vi "LoggingSpecificationDocument SetTestProperty.vi"(6 "contextId":T1, 8 "error in":errorcluster, 9 "timeout (ms)":i32=-1, 10 "Request Data":T3, 11 "gRPC ID":T1) -> (0 "error out":errorcluster, 2 "Response Data":T2, 3 "gRPC ID out":T1)   [LabVIEW 2020, in "FlexLogger_client.lvlib"]
uses:
  FlexLogger_client.lvlib
  <vilib>/gRPC/LabVIEW gRPC Library/Shared/grpcId.ctl
  RPC Messages/flexlogger_SetTestPropertyRequest.ctl
  RPC Messages/flexlogger_ElementIdentifier.ctl
  RPC Messages/flexlogger_TestProperty.ctl
  RPC Messages/flexlogger_SetTestPropertyResponse.ctl
  14035477-4c25-4107-8ed5-d0c4ef420ce5.vi
  <vilib>/gRPC/LabVIEW gRPC Library/Shared/TranslateGrpcError.vi
  <vilib>/gRPC/LabVIEW gRPC Library/Shared/Wait On Occurence.vi
  <vilib>/gRPC/LabVIEW gRPC Library/Server API/Server/Get Server DLL Path.vi
  <vilib>/Utility/error.llb/Error Cluster From Error Code.vi
  <vilib>/gRPC/LabVIEW gRPC Library/grpc-lvsupport-release.lvlib
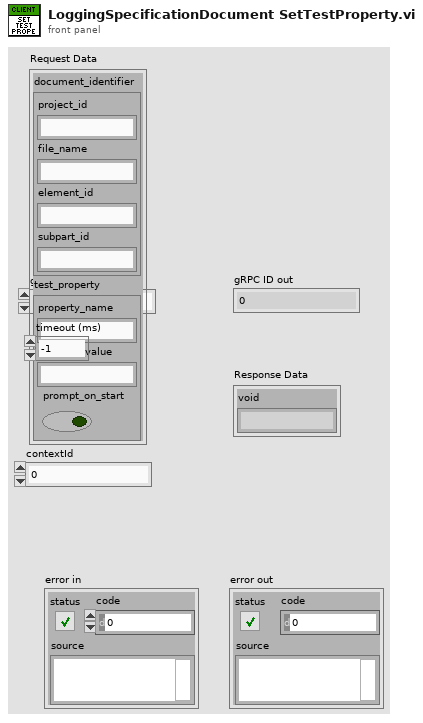
[diagram p1: front panel]
types:
  T1 = typedef "grpc-lvsupport-release.lvlib/grpcId.ctl" = u64
  T2 = typedef "FlexLogger_client.lvlib/flexlogger_SetTestPropertyResponse.ctl" = cluster{"void":string}
  T3 = typedef "FlexLogger_client.lvlib/flexlogger_SetTestPropertyRequest.ctl" = cluster{"document_identifier":T4, "test_property":T5}
  T4 = typedef "FlexLogger_client.lvlib/flexlogger_ElementIdentifier.ctl" = cluster{"project_id":string, "file_name":string, "element_id":string, "subpart_id":string}
  T5 = typedef "FlexLogger_client.lvlib/flexlogger_TestProperty.ctl" = cluster{"property_name":string, "property_value":string, "prompt_on_start":bool}
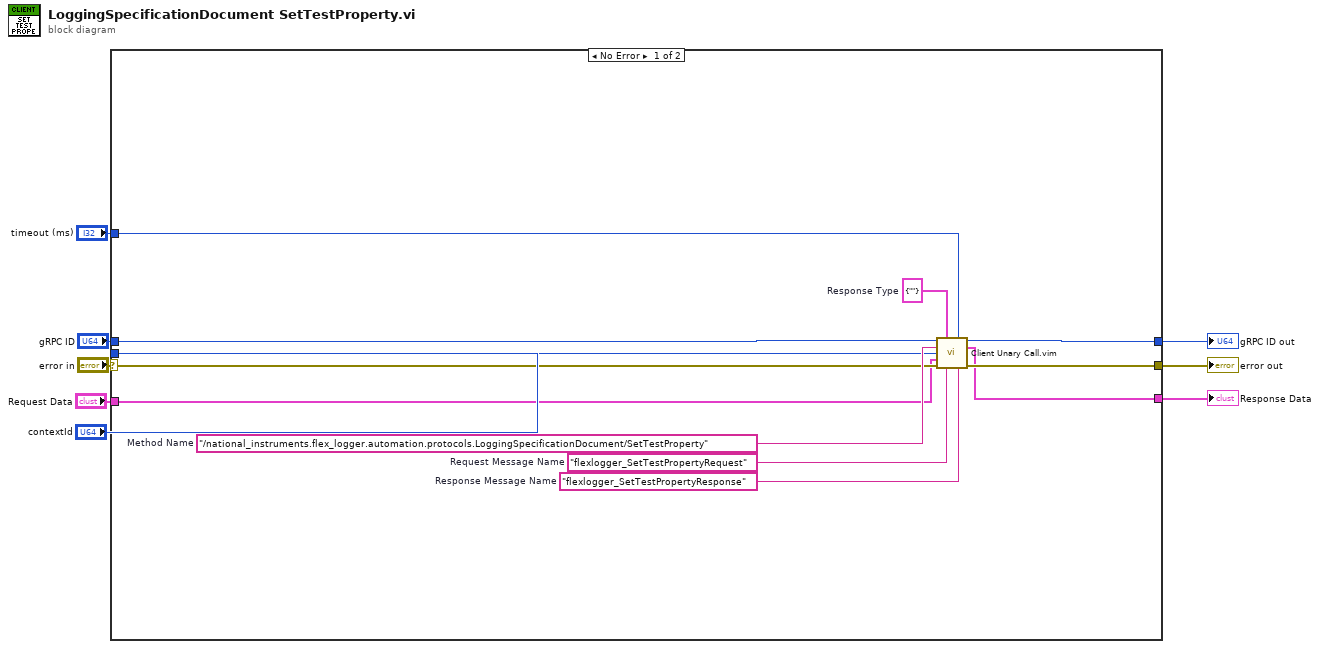
[diagram p0: block diagram]
diagram:
  n1 = case shown="No Error" "error in" {
    selector: "error in" -> [w16 w21]
    tunnel: [w15 w21] -> w7
    tunnel: "gRPC ID" -> [w14 w22]
    tunnel: [w13 w22] -> w5
    tunnel: "Request Data" -> [w12 _]
    tunnel: [w11 _] -> w3
    tunnel: "timeout (ms)" -> [w10 _]
    tunnel: "contextId" -> [w9 _]
    frame No Error {
      w17 = "flexlogger_SetTestPropertyResponse"  # Response Message Name
      w18 = "flexlogger_SetTestPropertyRequest"  # Request Message Name
      w19 = T2 {"void"=""}  # Response Type
      w20 = "/national_instruments.flex_logger.automation.protocols.LoggingSpecificationDocument/SetTestProperty"  # Method Name
      n2 = call "Client Unary Call.vim"("ClientID in"=w14, "Response Type"=w19, "timeout (ms)"=w10, "Method Name"=w20, "contextId"=w9, "Request Data"=w12, "error in"=w16, "Request Message Name"=w18, "Response Message Name"=w17) -> ("ClientID out"=w13:u64, "Response Data"=w11:T2, "error out"=w15:errorcluster)  [unwired: 4 in]
    }
    frame Error {
    }
  }
  "error out" <- w7
  "gRPC ID out" <- w5
  "Response Data" <- w3
